vi "Input.vi"(8 "error in (no error)":errorcluster, 9 "Dryer Control input":cluster{"Speed":dbl, "Temp":dbl, "Time":dbl}[](array[cluster]), 10 "Cluster":cluster{"Speed":u16, "Temp":u16, "Time":u16}, 11 "MASTER in":refnum<class "MASTER.lvclass">) -> (0 "error out":errorcluster, 3 "MASTER out":refnum<class "MASTER.lvclass">)   [LabVIEW 2014, in "Files Library.lvlib" / "MASTER.lvclass"]
uses:
  MASTER/MASTER.lvclass
  <vilib>/NI/Modbus Library/API/Master/Modbus Master.lvclass
panel:
  out "Recipe Indicator":string[][](array[string])
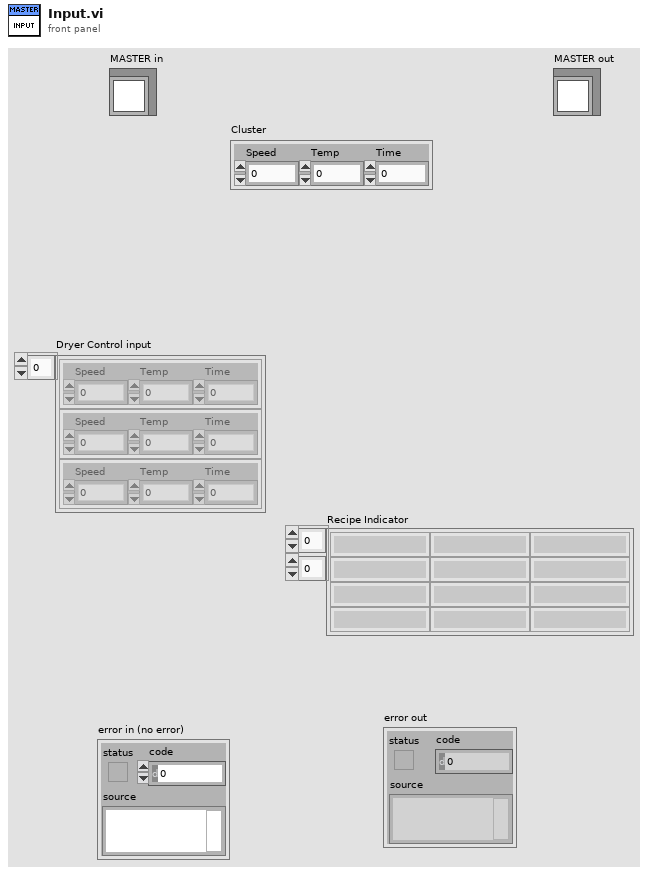
[diagram p1: front panel]
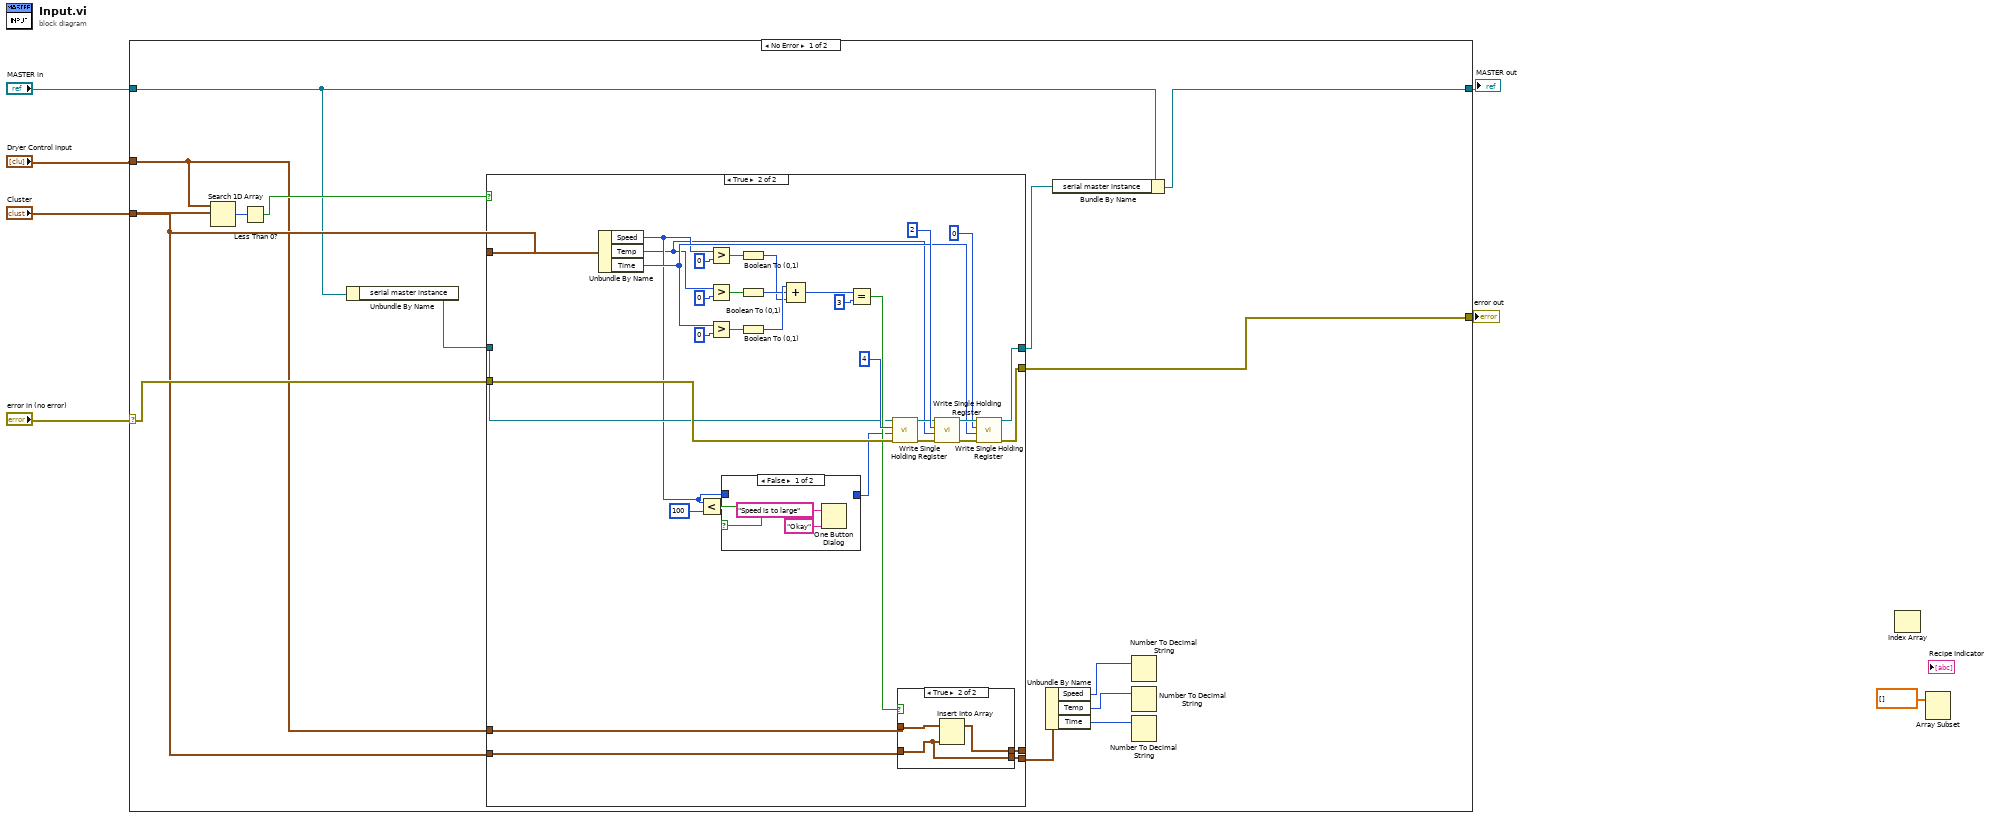
[diagram p0: block diagram]
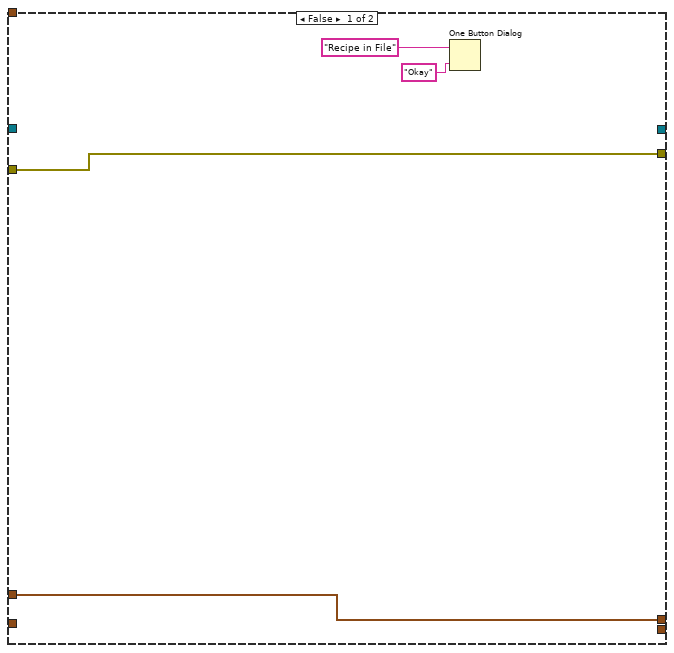
[diagram p2: hidden frame]
diagram:
  n1 = case shown="No Error" "error in (no error)" {
    selector: "error in (no error)" -> [w19 w69]
    tunnel: [w18 w69] -> w6
    tunnel: [w17 w68] -> w4
    tunnel: "MASTER in" -> [w13 w68]
    tunnel: "Dryer Control input" -> [w14 _]
    tunnel: "Cluster" -> [w15 _]
    frame No Error {
      n2 = Search 1D Array(1D array=w14, element=w15) -> (index of element=w21:i32)  [unwired: 1 in]
      n3 = Less Than 0?(x=w21) -> (x < 0?=w20:bool)
      n4 = Unbundle By Name(w13) -> ("serial master instance"=w12:refnum<class "Modbus Master.lvclass">)
      n5 = case shown="True" w20 {
        tunnel: w15 -> [_ w52]
        tunnel: w19 -> [w24 w51]
        tunnel: [w24 w50] -> w18
        tunnel: [_ w49] -> w16
        tunnel: w15 -> [_ w33]
        tunnel: [w25 w35] -> _
        tunnel: w14 -> [w25 w34]
        tunnel: w12 -> [_ w32]
        tunnel: [_ w26] -> w8
        frame False {
          n6 = One Button Dialog(message="Recipe in File", button name ("OK")="Okay") -> ()  [unwired: 1 out]
        }
        frame True {
          n7 = Unbundle By Name(w52) -> ("Speed"=w29:u16, "Temp"=w27:u16, "Time"=w45:u16)
          n8 = Less?(x=w29, y=u16 100) -> (x < y?=w30:bool)
          n9 = Greater?(x=w29, y=u16 0) -> (0:w44:bool)
          n10 = Greater?(x=w27, y=u16 0) -> (0:w43:bool)
          n11 = Greater?(x=w45, y=u16 0 ("Time")) -> (0:w42:bool)
          n12 = case shown="False" w30 {
            tunnel: [_ w62] -> w28
            tunnel: w29 -> [_ w62]
            frame False {
              n13 = One Button Dialog(message="Speed is to large", button name ("OK")="Okay") -> ()  [unwired: 1 out]
            }
            frame True {
            }
          }
          n14 = Boolean To (0,1)(Boolean=w44) -> (0, 1=w39:i16)
          n15 = Boolean To (0,1)(Boolean=w43) -> (0, 1=w40:i16)
          n16 = Boolean To (0,1)(Boolean=w42) -> (0, 1=w41:i16)
          n17 = Compound Arithmetic op=ADD(w41, w40, w39) -> (w37:i16)
          n18 = Equal?(x=w37, y=u16 3) -> (x = y?=w36:bool)
          n19 = call-dynamic "Write Single Holding Register.vi"("error in"=w51, "register to write"=w28, "address"=u16 4, "Modbus master in"=w32) -> ("error out"=w56:errorcluster, "Modbus master out"=w57:refnum<class "Modbus Master.lvclass">)  [unwired: 6 in]
          n20 = case shown="True" w36 {
            tunnel: [w64 w67] -> w35
            tunnel: w34 -> [w64 w66]
            tunnel: w33 -> [w63 w65]
            tunnel: [w63 w65] -> w26
            frame False {
            }
            frame True {
              n21 = Insert Into Array "Insert Into Array"(array=w66, new element=w65) -> (w67:cluster{"Speed":dbl, "Temp":dbl, "Time":dbl}[])  [unwired: 1 in]
            }
          }
          n22 = call-dynamic "Write Single Holding Register.vi"("error in"=w56, "register to write"=w27, "address"=u16 2, "Modbus master in"=w57) -> ("error out"=w54:errorcluster, "Modbus master out"=w55:refnum<class "Modbus Master.lvclass">)  [unwired: 6 in]
          n23 = call-dynamic "Write Single Holding Register.vi"("error in"=w54, "register to write"=w45, "address"=u16 0, "Modbus master in"=w55) -> ("error out"=w50:errorcluster, "Modbus master out"=w49:refnum<class "Modbus Master.lvclass">)  [unwired: 6 in]
        }
      }
      n24 = Unbundle By Name(w8) -> ("Speed"=w11:u16, "Temp"=w10:u16, "Time"=w9:u16)
      n25 = Bundle By Name(cluster=w13, "serial master instance"=w16) -> (w17:refnum<class "MASTER.lvclass">)
      n26 = Number To Decimal String(number=w11) -> ()  [unwired: 1 in, 1 out]
      n27 = Number To Decimal String(number=w10) -> ()  [unwired: 1 in, 1 out]
      n28 = Number To Decimal String(number=w9) -> ()  [unwired: 1 in, 1 out]
    }
    frame Error {
    }
  }
  "error out" <- w6
  "MASTER out" <- w4
  n29 = Index Array() -> ()  [unwired: 2 in, 1 out]
  n30 = Array Subset(array=dbl[] []) -> ()  [unwired: 2 in, 1 out]
